vi "Connect.vi"(8 "error in (no error)":errorcluster, 11 "Gantry In":refnum<k24>) -> (0 "error out":errorcluster, 3 "Gantry Out":refnum<k24>)   [LabVIEW 2019, in "A3200.lvclass"]
uses:
  A3200.lvclass
  C:/Program Files (x86)/Aerotech/A3200/LabVIEW/2010/Bin/Aerotech.A3200.dll
  Program Files (x86)/Aerotech/A3200/LabVIEW/2010/Bin/Aerotech.A3200.dll
  Drivers/Aerotech A3200/Aerotech VIs.lvlib
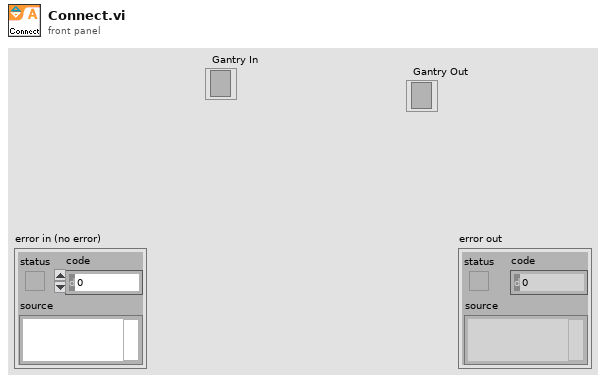
[diagram p1: front panel]
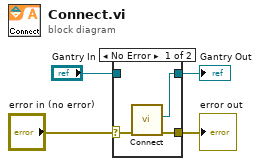
[diagram p0: block diagram]
diagram:
  n1 = case shown="No Error" "error in (no error)" {
    selector: "error in (no error)" -> [w6 w9]
    tunnel: [w5 w9] -> w3
    tunnel: "Gantry In" -> [_ w8]
    tunnel: [w7 w8] -> w1
    frame No Error {
      n2 = call "Connect.vi"("error in (no error)"=w6) -> ("error out"=w5:errorcluster, "controller"=w7:refnum<k24>)  [unwired: 9 in]
    }
    frame Error {
    }
  }
  "error out" <- w3
  "Gantry Out" <- w1
